vi "read_params.vi"(8 "error in (no error)":errorcluster, 11 "TruncatedSVD in":refnum<class "TruncatedSVD.lvclass">) -> (0 "error out":errorcluster, 2 "params":T1={"n_components"=2.0, "algorithm"="randomized", "n_iter"=5.0, "random_state"=0.0, "tol"=0.0}, 3 "TruncatedSVD out":refnum<class "TruncatedSVD.lvclass">)   [LabVIEW 2020, in "TruncatedSVD.lvclass"]
uses:
  TruncatedSVD.lvclass
  Controls/truncated_svd_params.ctl
  TruncatedSVD.lvclass/TruncatedSVD.ctl
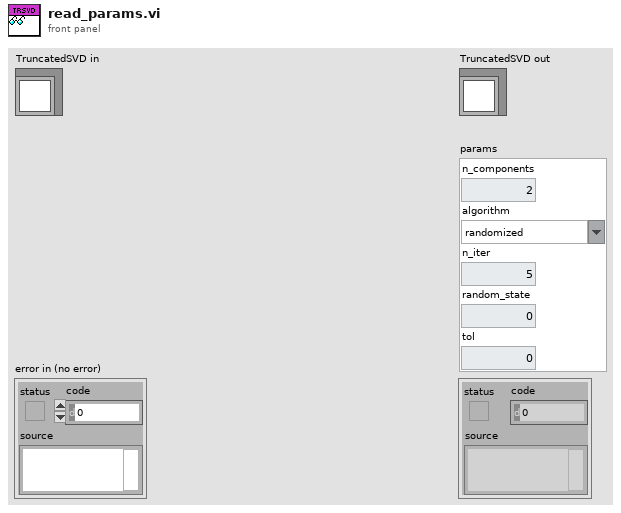
[diagram p1: front panel]
types:
  T1 = typedef "truncated_svd_params.ctl" = cluster{"n_components":dbl, "algorithm":string, "n_iter":dbl, "random_state":dbl, "tol":dbl}
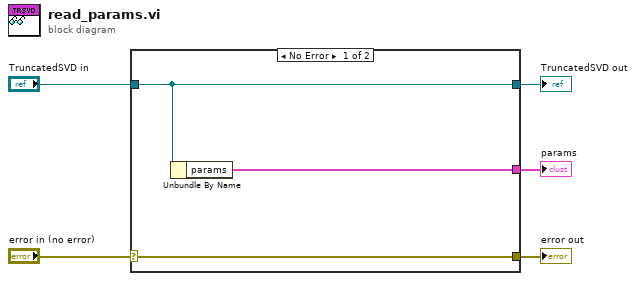
[diagram p0: block diagram]
diagram:
  n1 = case shown="No Error" "error in (no error)" {
    selector: "error in (no error)" -> [w8 w9]
    tunnel: [w8 w9] -> w4
    tunnel: [w7 w10] -> w2
    tunnel: "TruncatedSVD in" -> [w7 w10]
    tunnel: [w6 _] -> w1
    frame No Error {
      n2 = Unbundle By Name(w7) -> ("params"=w6:T1)
    }
    frame Error {
    }
  }
  "error out" <- w4
  "TruncatedSVD out" <- w2
  "params" <- w1
